vi "Teleop.vi"(10 "Match Info":T1={"Autonomous Elapsed Seconds"=0.0, "TeleOp Elapsed Seconds"=0.0, "Disabled Elapsed Seconds"=0.0, "Visited Autonomous"=FALSE, "Visited TeleOp"=FALSE, "Visited Disabled"=FALSE, "Autonomous Settings"={"Autonomous Style"=enum."Independent", "VI Refnum"=refnum}}, 11 "Call Context":T2) -> ()   [LabVIEW 2019]
doc: "This VI is called for each TeleOp packet received from the DS where the robot is not disabled. It is often used to read from the joysticks and update I/O or to update setpoints for timed control loops. It should complete and return within 20 milliseconds or it may miss DS packets."
uses:
  <vilib>/Rock Robotics/WPI/DriverStation/WPI_DriverStationDerivedRobotMode.ctl
  <vilib>/Rock Robotics/WPI/DriverStation/WPI_DriverStationMatch Info.ctl
  <vilib>/Rock Robotics/WPI/Utilities/WPI_GetSetVariantRefNum.vi
  Driver Globals.vi
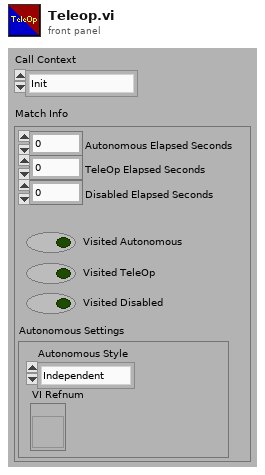
[diagram p1: front panel]
types:
  T1 = typedef "WPI_DriverStationMatch Info.ctl" = cluster{"Autonomous Elapsed Seconds":dbl, "TeleOp Elapsed Seconds":dbl, "Disabled Elapsed Seconds":dbl, "Visited Autonomous":bool, "Visited TeleOp":bool, "Visited Disabled":bool, "Autonomous Settings":cluster{"Autonomous Style":enum16{"Iterative", "Independent"}, "VI Refnum":refnum<vi>}}
  T2 = typedef "WPI_DriverStationDerivedRobotMode.ctl" = enum16{"Init", "Execute", "Stop"}
  T3 = typedef "WPI_JoystickDevRef.ctl" = cluster{"Device":T4}
  T4 = typedef "WPI_JoystickDeviceEnum.ctl" = enum16{"USB 0", "USB 1", "USB 2", "USB 3", "USB 4", "USB 5"}
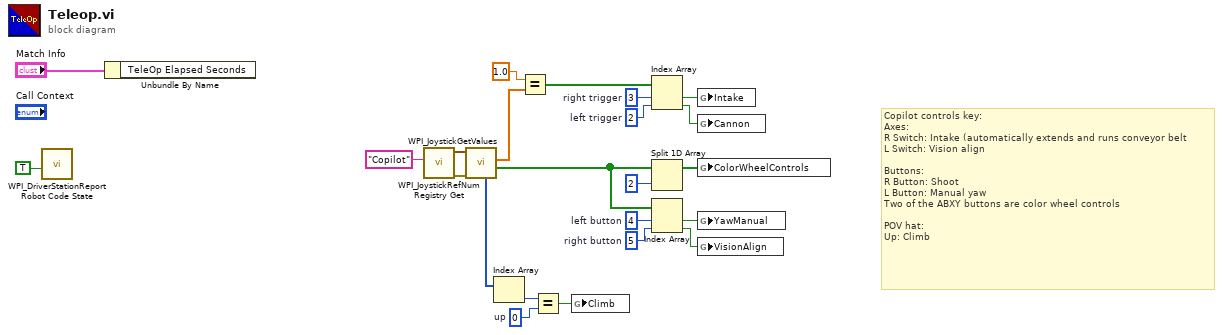
[diagram p0: block diagram]
diagram:
  w3 = i16 0  # up
  w14 = 5  # right button
  w15 = 4  # left button
  w16 = 2  # left trigger
  w17 = 3  # right trigger
  # "Copilot controls key:\nAxes:\nR Switch: Intake (automatically extends and runs conveyor belt\nL Switch: Vision align\n\nButtons:\nR Button: Shoot\nL Button: Manual yaw\nTwo of the ABXY buttons are color wheel controls\n\nPOV hat:\nUp: Climb"
  n1 = call <vilib>:"WPI_DriverStationReport Robot Code State.vi"("TeleOp"=TRUE ("Autonomous")) -> ()  [unwired: 10 in, 1 out]
  n2 = Unbundle By Name("Match Info") -> ()  [unwired: 1 out]
  n3 = call <vilib>:"WPI_JoystickRefNum Registry Get.vi"("refnum name"="Copilot") -> ("error out"=w19:errorcluster, "JoystickDevRef"=w20:T3)  [unwired: 9 in]
  n4 = call <vilib>:"WPI_JoystickGetValues.vi"("error in (no error)"=w19, "JoystickDevRef"=w20) -> ("Buttons"=w11:bool[], "Axes"=w18:dbl[], "POVs"=w5:i16[])  [unwired: 5 in, 2 out]
  n5 = Index Array(array=w5) -> (element=w4:i16)  [unwired: 1 in]
  n6 = Equal?(x=1.0, y=w18) -> (x = y?=w8:bool[])
  n7 = Equal?(x=w4, y=w3) -> (x = y?=w2:bool)
  n8 = global write "Driver Globals.vi" "Climb"(w2) -> ()
  n9 = Index Array(array=w8, index #1=w17, index #2=w16) -> (element #1=w6:bool, element #2=w1:bool)
  n10 = Split 1D Array(array=w11, index=2) -> (first subarray=w12:bool[])  [unwired: 1 out]
  n11 = Index Array(array=w11, index #1=w15, index #2=w14) -> (element #1=w10:bool, element #2=w9:bool)
  n12 = global write "Driver Globals.vi" "Intake"(w6) -> ()
  n13 = global write "Driver Globals.vi" "Cannon"(w1) -> ()
  n14 = global write "Driver Globals.vi" "ColorWheelControls"(w12) -> ()
  n15 = global write "Driver Globals.vi" "YawManual"(w10) -> ()
  n16 = global write "Driver Globals.vi" "VisionAlign"(w9) -> ()
